vi "4461 + sync pulse demo.vi"() -> ()   [LabVIEW 2015]
uses:
  <vilib>/DAQmx/write.llb/DAQmx Write (Analog 1D DBL 1Chan NSamp).vi
  <vilib>/DAQmx/create/channels.llb/DAQmx Create Channel (AO-Voltage-Basic).vi
  <vilib>/DAQmx/configure/timing.llb/DAQmx Timing (Sample Clock).vi
  <vilib>/DAQmx/miscellaneous.llb/DAQmx Fill In Error Info.vi
  <vilib>/DAQmx/create/channels.llb/DAQmx Create Channel (CO-Pulse Generation-Ticks).vi
  <vilib>/DAQmx/configure/timing.llb/DAQmx Timing (Implicit).vi
  <vilib>/DAQmx/configure/trigger.llb/DAQmx Start Trigger (Digital Edge).vi
  <resource>/objmgr/daqmx.rc
  <vilib>/Analysis/NI_AALBase.lvlib
panel:
  in  "stop":bool
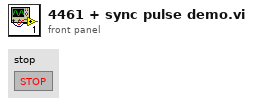
[diagram p1: front panel]
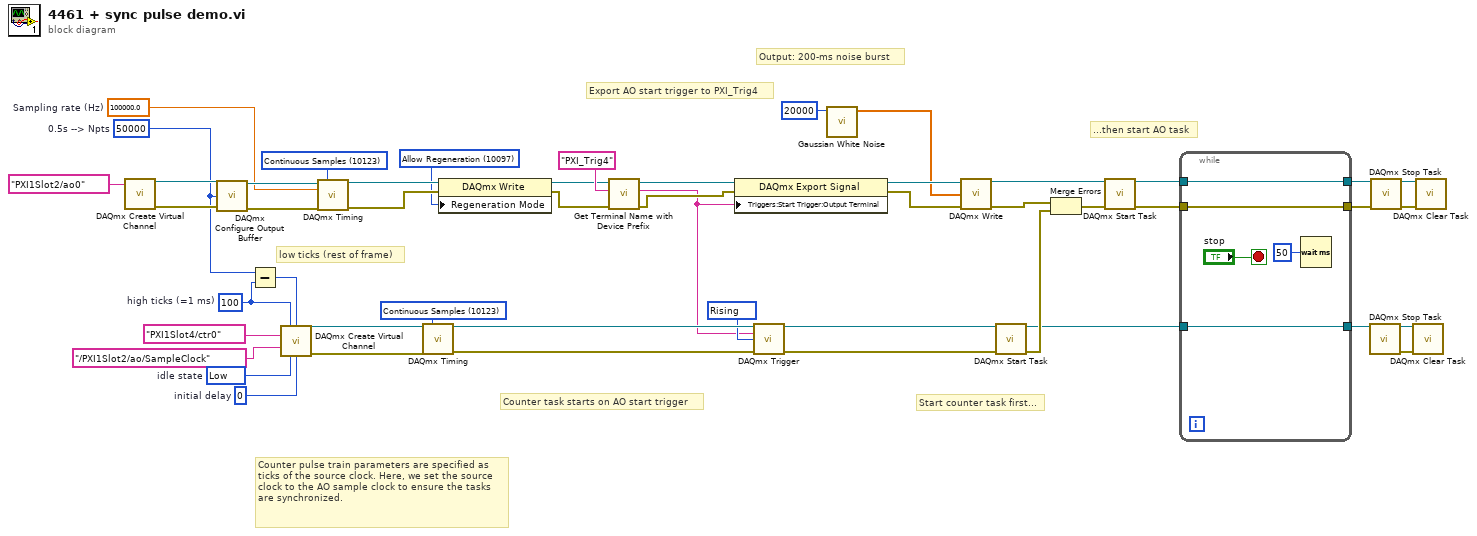
[diagram p0: block diagram]
diagram:
  w9 = 10280 items=["Rising"=10280, "Falling"=10171] ("Trigger Edge")
  w8 = 10123 items=["Finite Samples"=10178, "Continuous Samples"=10123] ("sample mode")
  w12 = u32 0  # initial delay
  w13 = 10214 items=["High"=10192, "Low"=10214]  # idle state
  w15 = u32 100  # high ticks (=1 ms)
  w21 = 100000.0  # Sampling rate (Hz)
  w16 = 50000  # 0.5s --> Npts
  w41 = 10123 items=["Finite Samples"=10178, "Continuous Samples"=10123, "Hardware Timed Single Point"=12522] ("sample mode")
  w45 = 10097 items=["Allow Regeneration"=10097, "Do Not Allow Regeneration"=10158] ("RegenMode")
  # "Counter pulse train parameters are specified as ticks of the source clock. Here, we set the source clock to the AO sample clock to ensure the tasks are synchronized."
  # "Export AO start trigger to PXI_Trig4"
  # "...then start AO task"
  # "Start counter task first..."
  # "Counter task starts on AO start trigger"
  # "low ticks (rest of frame)"
  # "Output: 200-ms noise burst"
  n1 = call-poly <vilib>:"DAQmx Create Virtual Channel.vi"("physical channels"=tag "PXI1Slot2/ao0") -> ("task out"=w49:refnum<k21>, "error out"=w44:errorcluster)  [unwired: 13 in]
  n2 = call <vilib>:"DAQmx Configure Output Buffer.vi"("task/channels in"=w49, "buffer size (in samples per channel)"=w16, "error in"=w44) -> ("task out"=w48:refnum<k21>, "error out"=w43:errorcluster)  [unwired: 11 in]
  n3 = Subtract(x=w16, y=w15) -> (x-y=w14:u32)
  n4 = call-poly <vilib>:"DAQmx Create Virtual Channel.vi"("high ticks"=w15, "low ticks"=w14, "counter"=tag "PXI1Slot4/ctr0", "source of ticks"=tag "/PXI1Slot2/ao/SampleClock", "idle state"=w13, "initial delay"=w12) -> ("task out"=w7:refnum<k21>, "error out"=w6:errorcluster)  [unwired: 8 in]
  n5 = call-poly <vilib>:"DAQmx Timing.vi"("task/channels in"=w48, "sample mode"=w41, "rate"=w21, "error in"=w43) -> ("task out"=w46:refnum<k21>, "error out"=w47:errorcluster)  [unwired: 10 in]
  n6 = call-poly <vilib>:"DAQmx Timing.vi"("task/channels in"=w7, "sample mode"=w8, "error in"=w6) -> ("task out"=w10:refnum<k21>, "error out"=w11:errorcluster)  [unwired: 11 in]
  n7 = property class="DAQmx Write"(reference=w46, error in=w47, "Regeneration Mode"=w45) -> (reference out=w37:refnum<k21>, error out=w36:errorcluster)
  n8 = call "Get Terminal Name with Device Prefix.vi"("error in (no error)"=w36, "Local Terminal Name"="PXI_Trig4", "task/channels in"=w37) -> ("error out"=w39:errorcluster, "Terminal Name with Device Prefix"=w5:tag, "task out"=w38:refnum<k21>)  [unwired: 6 in]
  n9 = property class="DAQmx Export Signal"(reference=w38, error in=w39, "Triggers:Start Trigger:Output Terminal"=w5) -> (reference out=w25:refnum<k21>, error out=w23:errorcluster)
  n10 = call-poly <vilib>:"DAQmx Trigger.vi"("task/channels in"=w10, "source"=w5, "edge"=w9, "error in"=w11) -> ("task out"=w2:refnum<k21>, "error out"=w1:errorcluster)  [unwired: 10 in]
  n11 = call <vilib>:"Gaussian White Noise.vi"("samples"=20000) -> ("Gaussian noise pattern"=w19:dbl[])  [unwired: 9 in, 1 out]
  n12 = call-poly <vilib>:"DAQmx Write.vi"("task/channels in"=w25, "data"=w19, "error in"=w23) -> ("task out"=w24:refnum<k21>, "error out"=w22:errorcluster)  [unwired: 10 in, 1 out]
  n13 = call <vilib>:"DAQmx Start Task.vi"("task/channels in"=w2, "error in"=w1) -> ("task out"=w31:refnum<k21>, "error out"=w35:errorcluster)  [unwired: 12 in]
  n14 = Merge Errors(w22, w35) -> (w34:errorcluster)
  n15 = call <vilib>:"DAQmx Start Task.vi"("task/channels in"=w24, "error in"=w34) -> ("task out"=w32:refnum<k21>, "error out"=w33:errorcluster)  [unwired: 12 in]
  n16 = while {
    tunnel: w33 -> [w51]
    tunnel: w32 -> [w52]
    tunnel: w31 -> [w50]
    tunnel: [w52] -> w30
    tunnel: [w51] -> w29
    tunnel: [w50] -> w28
    stop <- "stop" stop-if-true
    n17 = Wait (ms)(milliseconds to wait=u32 50) -> ()  [unwired: 1 out]
  }
  n18 = call <vilib>:"DAQmx Stop Task.vi"("task/channels in"=w28) -> ("task out"=w4:refnum<k21>, "error out"=w3:errorcluster)  [unwired: 13 in]
  n19 = call <vilib>:"DAQmx Stop Task.vi"("task/channels in"=w30, "error in"=w29) -> ("task out"=w27:refnum<k21>, "error out"=w26:errorcluster)  [unwired: 12 in]
  n20 = call <vilib>:"DAQmx Clear Task.vi"("task in"=w4, "error in"=w3) -> ()  [unwired: 13 in, 1 out]
  n21 = call <vilib>:"DAQmx Clear Task.vi"("task in"=w27, "error in"=w26) -> ()  [unwired: 13 in, 1 out]
